vi "group Bulk Write Remove Param.vi"(10 "id":u8, 11 "group_num":i32) -> ()   [LabVIEW 2015, in "dxl_x86_c.lvlib"]
doc: "WINDECLSPEC void groupBulkWriteRemoveParam (int group_num, uint8_t id);"
uses:
  dxl_x86_c.lvlib
  dxl_x86_c.dll
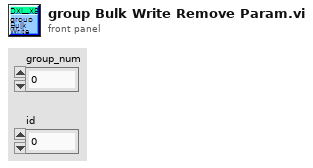
[diagram p1: front panel]
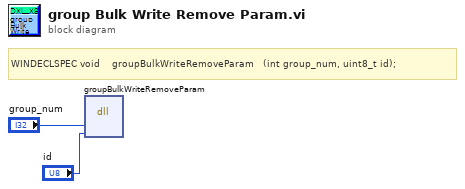
[diagram p0: block diagram]
diagram:
  # "WINDECLSPEC void    groupBulkWriteRemoveParam   (int group_num, uint8_t id);"
  n1 = dll-call lib="C:/Users/Platform/Desktop/LabVIEW/dxl_x86_c.lvlib/dxl_x86_c.*" fn="groupBulkWriteRemoveParam"("group_num"="group_num", "id"="id") -> ()  [unwired: 6 in, 2 out]
